vi "BPSK_AddSync.vi"(5 "Preamble":dbl[](array[numeric]), 8 "error in (no error)":errorcluster caption="错误输入（无错误）", 10 "Channel_Bit":dbl[](array[numeric]) format="%#_13g", 11 "PathIn":path) -> (0 "error out":errorcluster caption="错误输出", 2 "data":dbl[](array[numeric]), 3 "PathOut":path)   [LabVIEW 2015]
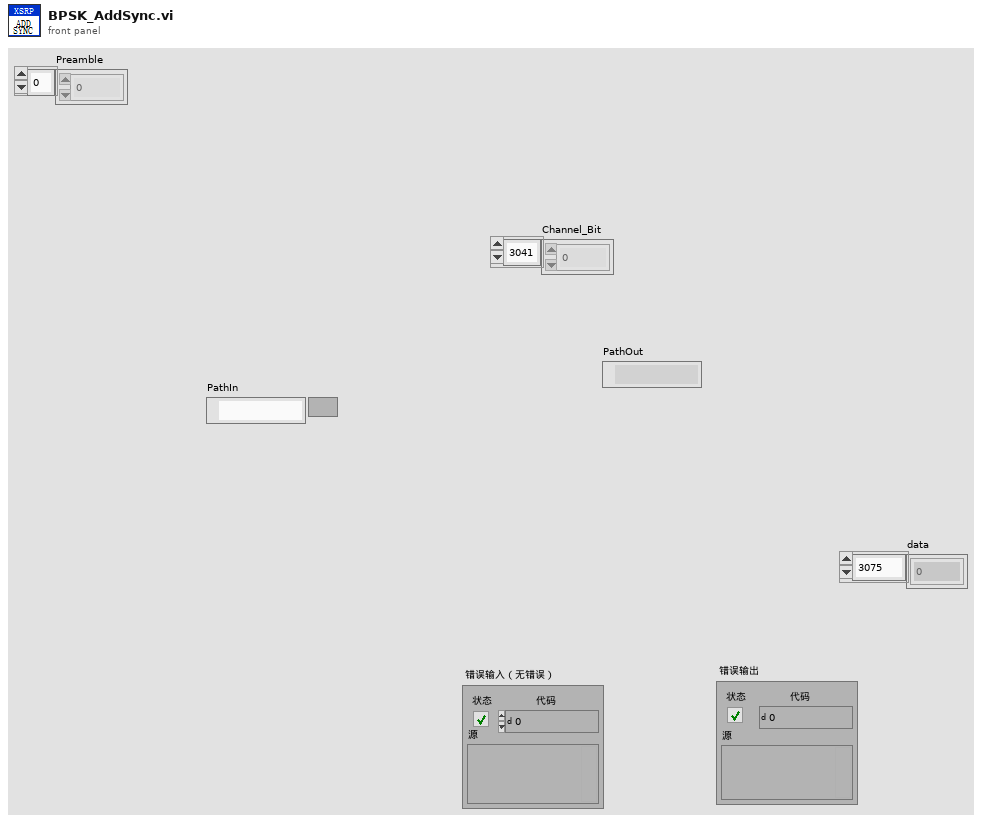
[diagram p1: front panel]
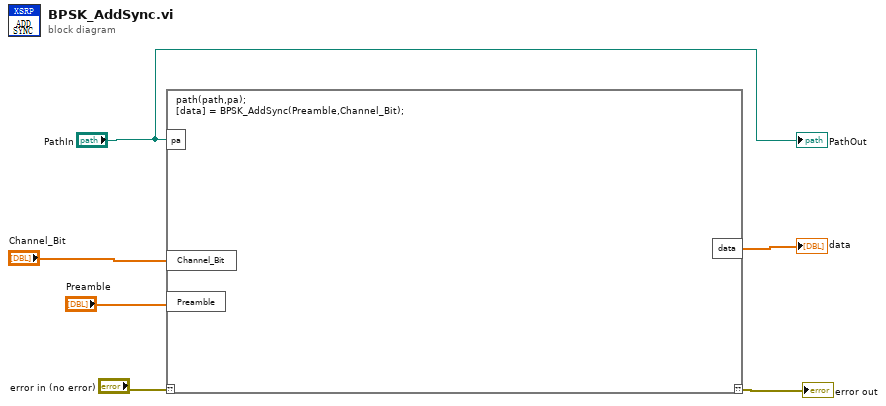
[diagram p0: block diagram]
diagram:
  n1 = script code="path(path,pa);\n[data] = BPSK_AddSync(Preamble,Channel_Bit);"("??"="error in (no error)", "pa"="PathIn", "Channel_Bit"="Channel_Bit", "Preamble"="Preamble") -> ("??"=→"error out":errorcluster, "data"=→"data":dbl[])
  "PathOut" <- "PathIn"
